vi "Delay.vi"(0 "Enable?":bool, 2 "Delay":dbl) -> (4 "Output":bool)   [LabVIEW 2016]
uses:
  Change Detect Boolean.vi
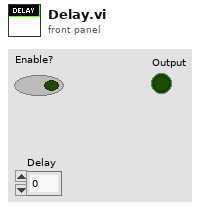
[diagram p1: front panel]
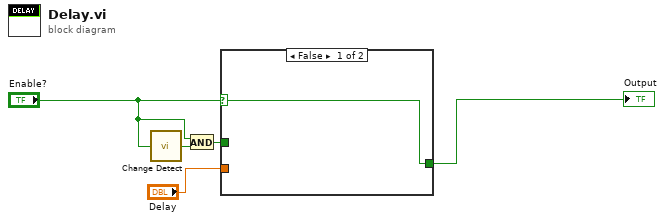
[diagram p0: block diagram]
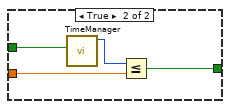
[diagram p2: hidden frame]
diagram:
  n1 = call-poly "Change Detect.vi"("In"="Enable?") -> ("Changed?"=w5:bool)
  n2 = And(x="Enable?", y=w5) -> (x .and. y?=w2:bool)
  n3 = case shown="False" "Enable?" {
    selector: "Enable?" -> [w6 _]
    tunnel: w2 -> [_ w10]
    tunnel: "Delay" -> [_ w8]
    tunnel: [w6 w7] -> w3
    frame False {
    }
    frame True {
      n4 = call "TimeManager.vi"("Reset?"=w10) -> ("Time Since Reset"=w9:u32)  [unwired: 9 in, 1 out]
      n5 = Less Or Equal?(x=w9, y=w8) -> (x <= y?=w7:bool)
    }
  }
  "Output" <- w3
